vi "Set ni_measurementlink_measurement_v1_MeasureResponse.vi"(7 "Complete Call (T)":bool=TRUE, 8 "error in (no error)":errorcluster, 10 "package_templatemessage":T1, 11 "gRPCid":T3) -> (0 "error out":errorcluster)   [LabVIEW 2021, in "ni.measurementlink.measurement.v1.api.lvlib"]
uses:
  ni.measurementlink.measurement.v1.api.lvlib
  <vilib>/gRPC/LabVIEW gRPC Library/Shared/grpcId.ctl
  ni_measurementlink_measurement_v1_MeasureResponse.ctl
  google_protobuf_Any.ctl
  ni_measurementlink_measurement_v1_MeasureResponse_Flat.ctl
  google_protobuf_Any_Flat.ctl
  dcc74a39-081a-4bdd-860b-8ed792803c96.vi
  <vilib>/gRPC/LabVIEW gRPC Library/Shared/TranslateGrpcError.vi
  RichToFlatgoogle_protobuf_Any.vi
  <vilib>/gRPC/LabVIEW gRPC Library/Server API/Server/Get Server DLL Path.vi
  <vilib>/Utility/error.llb/Error Cluster From Error Code.vi
  <vilib>/gRPC/LabVIEW gRPC Library/grpc-lvsupport-release.lvlib
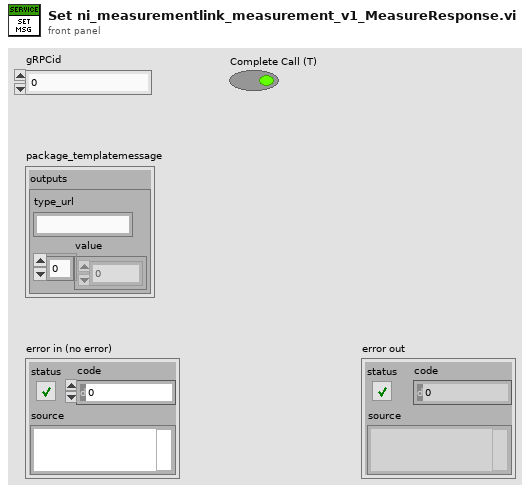
[diagram p1: front panel]
types:
  T1 = typedef "ni.measurementlink.measurement.v1.api.lvlib/ni_measurementlink_measurement_v1_MeasureResponse.ctl" = cluster{"outputs":T2}
  T2 = typedef "ni.measurementlink.measurement.v1.api.lvlib/google_protobuf_Any.ctl" = cluster{"type_url":string, "value":u8[]}
  T3 = typedef "grpc-lvsupport-release.lvlib/grpcId.ctl" = u64
  T4 = typedef "ni.measurementlink.measurement.v1.api.lvlib/ni_measurementlink_measurement_v1_MeasureResponse_Flat.ctl" = cluster{"outputs":T5}
  T5 = typedef "ni.measurementlink.measurement.v1.api.lvlib/google_protobuf_Any_Flat.ctl" = cluster{"type_url":string, "value":u8[]}
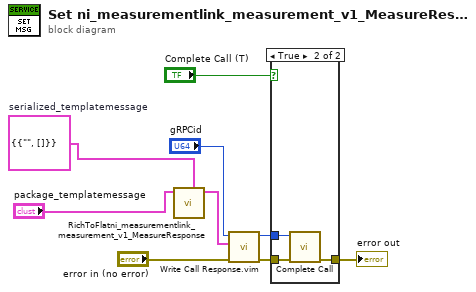
[diagram p0: block diagram]
diagram:
  w2 = T4 {"outputs"={"type_url"="", "value"=[]}}  # serialized_templatemessage
  n1 = call "RichToFlatni_measurementlink_measurement_v1_MeasureResponse.vi"("OutputClusterType"=w2, "InputCluster"="package_templatemessage") -> ("OutputCluster"=w1:T4)  [unwired: 9 in]
  n2 = call "Write Call Response.vim"("error in"="error in (no error)", "Response Data"=w1, "gRPCid in"="gRPCid") -> ("error out"=w6:errorcluster, "gRPCid out"=w7:T3)  [unwired: 7 in]
  n3 = case shown="True" "Complete Call (T)" {
    tunnel: [w10 w13] -> w9
    tunnel: w7 -> [_ w12]
    tunnel: w6 -> [w10 w11]
    frame False {
    }
    frame True {
      n4 = call <vilib>:"Complete Call.vi"("gRPCid"=w12, "error in"=w11) -> ("error out"=w13:errorcluster)  [unwired: 8 in]
    }
  }
  "error out" <- w9
